vi "FGV_ExclusionList_Manager.vi"(7 "Actions":T1, 8 "error in (no error)":errorcluster, 11 "XML 2D Array":string[][](array[string])) -> (0 "error out":errorcluster, 1 "To Exclude":string[][](array[string]), 2 "To Include":string[][](array[string]), 3 "Exclusion Params (from  file)":string[][](array[string]), 4 "Channel Paths":string[][](array[string]), 5 "Objective Paths":string[][](array[string]))   [LabVIEW 2012]
doc: "SciScan 1.2 160622"
uses:
  FGV_ExclusionList_Manager_Commands.ctl
  <vilib>/Utility/file.llb/Read From Spreadsheet File (string).vi
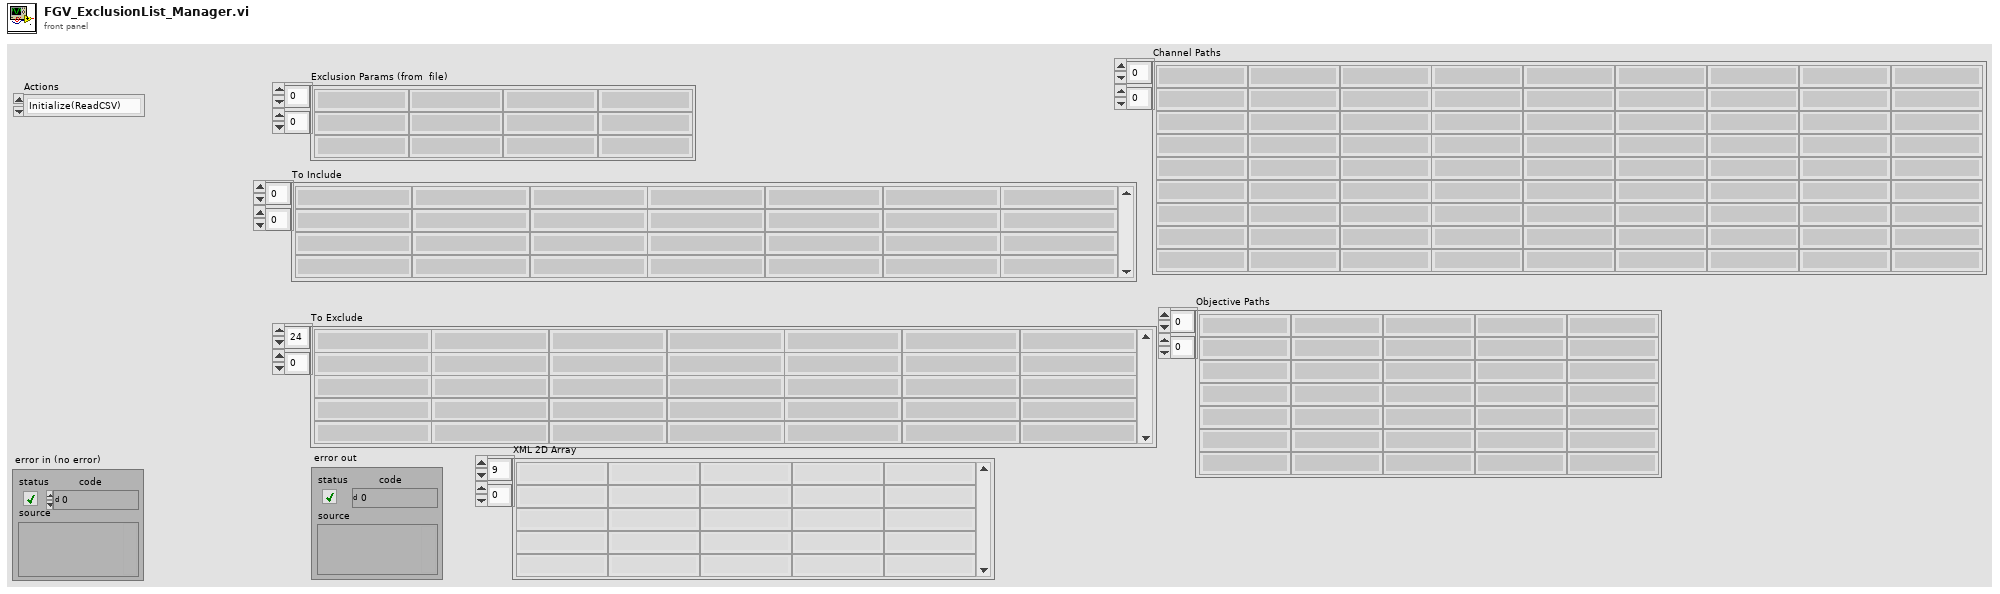
[diagram p1: front panel]
types:
  T1 = typedef "FGV_ExclusionList_Manager_Commands.ctl" = enum16{"Initialize(ReadCSV)", "Get", "CategorizePaths"}
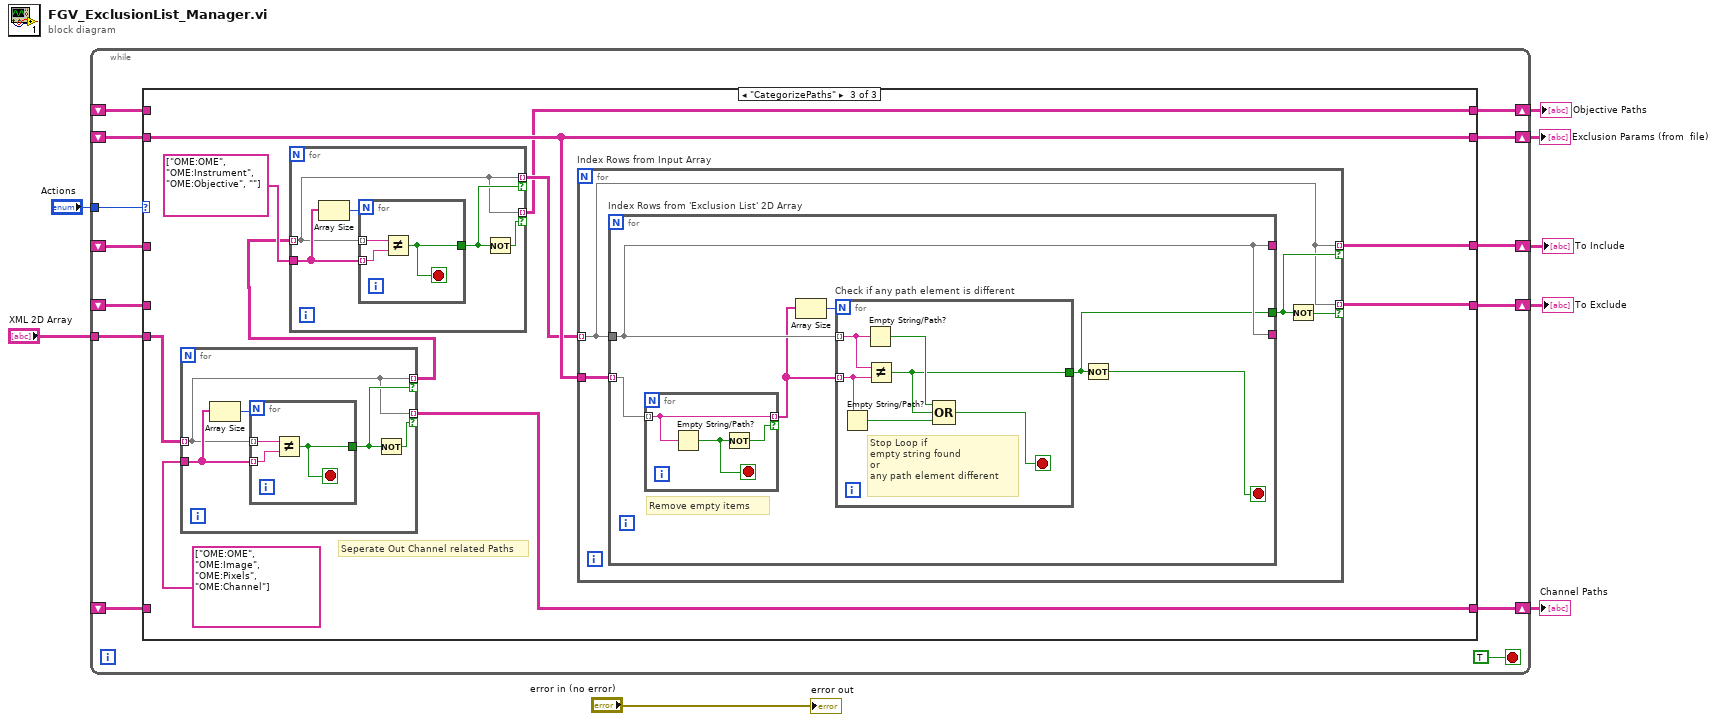
[diagram p0: block diagram]
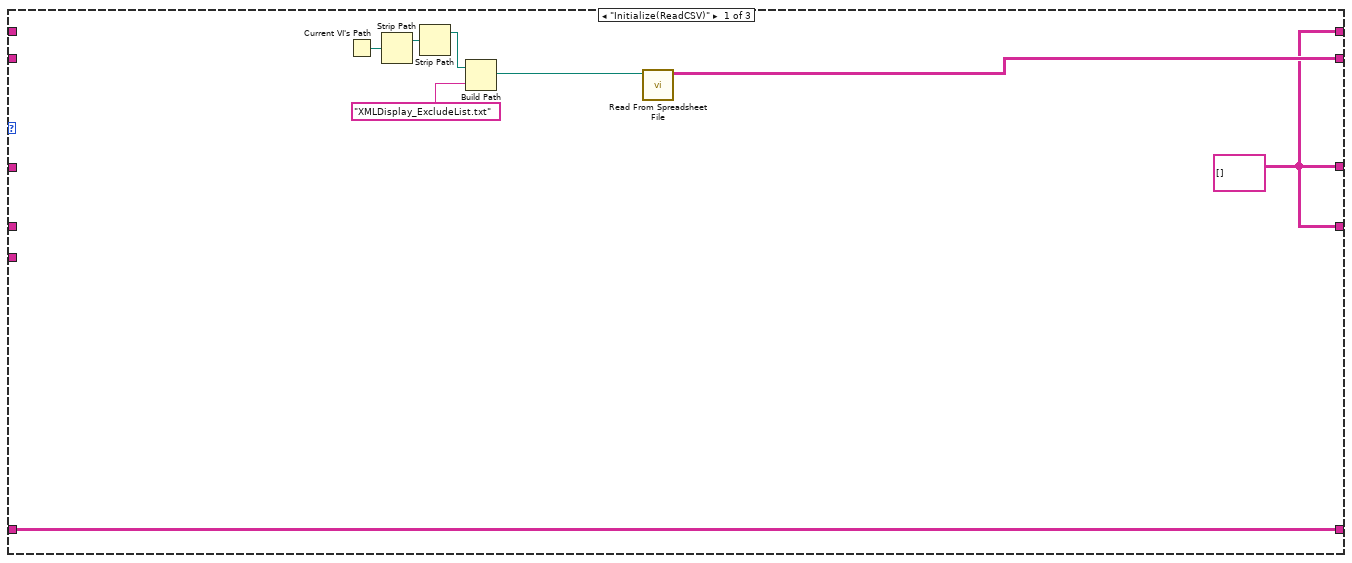
[diagram p2: hidden frame]
diagram:
  n1 = while {
    tunnel: "Actions" -> [w21]
    shift-right: [w19] -> w7
    shift-left: _ -> [w18]
    tunnel: "XML 2D Array" -> [w17]
    shift-right: [w16] -> w3
    shift-left: _ -> [w14]
    shift-right: [w15] -> w4
    shift-left: _ -> [w13]
    shift-right: [w12] -> w2
    shift-left: _ -> [w11]
    shift-right: [w10] -> w1
    shift-left: _ -> [w9]
    stop <- TRUE stop-if-true
    n2 = case shown="\"CategorizePaths\"" w21 {
      tunnel: [w24 w34 w44] -> w19
      tunnel: w18 -> [_ w34 w44]
      tunnel: w17 -> [_ _ w39]
      tunnel: [w22 w32 w43] -> w16
      tunnel: [w22 w33 w42] -> w15
      tunnel: w14 -> [_ w32 _]
      tunnel: w13 -> [_ w33 _]
      tunnel: [w23 w31 w40] -> w12
      tunnel: w11 -> [w23 w31 _]
      tunnel: [w22 w30 w35] -> w10
      tunnel: w9 -> [_ w30 _]
      frame "Initialize(ReadCSV)" {
        w22 = string[][] [] ("XML 2D Array")
        n3 = Current VI's Path() -> (path=w29:path)
        n4 = Strip Path(path=w29) -> (stripped path=w28:path)  [unwired: 1 out]
        n5 = Strip Path(path=w28) -> (stripped path=w27:path)  [unwired: 1 out]
        n6 = Build Path(base path=w27, name or relative path="XMLDisplay_ExcludeList.txt") -> (appended path=w25:path)
        n7 = call-poly <vilib>:"Read From Spreadsheet File.vi"("file path (dialog if empty)"=w25) -> ("all rows"=w24:string[][])  [unwired: 6 in, 4 out]
      }
      frame "Get", Default {
      }
      frame "CategorizePaths" {
        # "Seperate Out Channel related Paths"
        n8 = for {
          tunnel: w39 -> [w54] mode=indexing
          tunnel: string[] ["OME:OME", "OME:Image", "OME:Pixels", "OME:Channel"] ("To Exclude") -> [w57]
          tunnel: [w54] -> w37 mode=indexing if=w55
          tunnel: [w54] -> w40 mode=indexing if=w53
          n9 = Array Size(array=w57) -> (size(s)=w56:i32)
          n10 = for {
            N: w56 -> [_]
            tunnel: w57 -> [w59] mode=indexing
            tunnel: w54 -> [w60] mode=indexing
            tunnel: [w58] -> w55
            stop <- w58 stop-if-true
            n11 = Not Equal?(x=w60, y=w59) -> (x != y?=w58:bool)
          }
          n12 = Not(x=w55) -> (.not. x?=w53:bool)
        }
        n13 = for {
          tunnel: w37 -> [w46] mode=indexing
          tunnel: string[] ["OME:OME", "OME:Instrument", "OME:Objective", ""] ("To Exclude") -> [w49]
          tunnel: [w46] -> w36 mode=indexing if=w47
          tunnel: [w46] -> w35 mode=indexing if=w45
          n14 = Array Size(array=w49) -> (size(s)=w48:i32)
          n15 = for {
            N: w48 -> [_]
            tunnel: w49 -> [w51] mode=indexing
            tunnel: w46 -> [w52] mode=indexing
            tunnel: [w50] -> w47
            stop <- w50 stop-if-true
            n16 = Not Equal?(x=w52, y=w51) -> (x != y?=w50:bool)
          }
          n17 = Not(x=w47) -> (.not. x?=w45:bool)
        }
        n18 = for "Index Rows from Input Array" {
          tunnel: w36 -> [w61] mode=indexing
          tunnel: w44 -> [w64]
          tunnel: [w61] -> w42 mode=indexing if=w63
          tunnel: [w61] -> w43 mode=indexing if=w62
          n19 = for "Index Rows from 'Exclusion List' 2D Array" {
            tunnel: w61 -> [w70]
            tunnel: w64 -> [w66] mode=indexing
            tunnel: [w70] -> _
            tunnel: [w70] -> _
            tunnel: [w67] -> w63
            stop <- w68 stop-if-true
            # "Remove empty items"
            n20 = for {
              tunnel: w66 -> [w73] mode=indexing
              tunnel: [w73] -> w65 mode=indexing if=w72
              stop <- w71 stop-if-true
              n21 = Empty String/Path?(string/path=w73) -> (empty?=w71:bool)
              n22 = Not(x=w71) -> (.not. x?=w72:bool)
            }
            n23 = Array Size(array=w65) -> (size(s)=w69:i32)
            n24 = for "Check if any path element is different" {
              N: w69 -> [_]
              tunnel: w65 -> [w78] mode=indexing
              tunnel: w70 -> [w79] mode=indexing
              tunnel: [w75] -> w67
              stop <- w74 stop-if-true
              # "Stop Loop if\nempty string found\nor\nany path element different"
              n25 = Empty String/Path?(string/path=w78) -> (empty?=w77:bool)
              n26 = Empty String/Path?(string/path=w79) -> (empty?=w76:bool)
              n27 = Not Equal?(x=w79, y=w78) -> (x != y?=w75:bool)
              n28 = Compound Arithmetic op=OR(w76, w75, w77) -> (w74:bool)
            }
            n29 = Not(x=w67) -> (.not. x?=w68:bool)
          }
          n30 = Not(x=w63) -> (.not. x?=w62:bool)
        }
      }
    }
  }
  "Exclusion Params (from  file)" <- w7
  "To Exclude" <- w3
  "To Include" <- w4
  "Channel Paths" <- w2
  "Objective Paths" <- w1
  "error out" <- "error in (no error)"
